vi "UPQLTY.vi"(0 "工位追溯码":string, 1 "检测项目":string, 2 "单位":string, 3 "检测值":string, 4 "检测结果":string, 5 "错误输入":errorcluster, 6 "总成追溯码":string, 7 "设备编号":string, 8 "操作员":string, 9 "产品型号":string, 11 "标准值":string) -> (19 "error out":errorcluster)   [LabVIEW 2020]
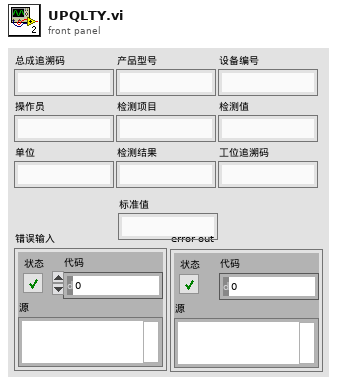
[diagram p1: front panel]
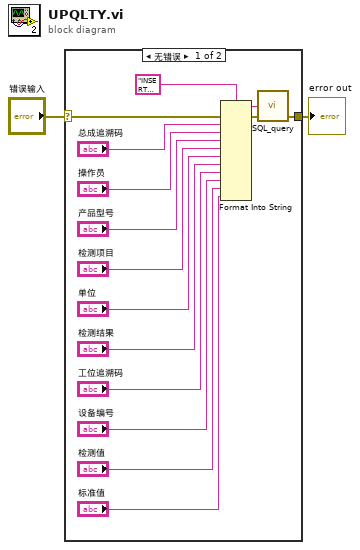
[diagram p0: block diagram]
diagram:
  n1 = case shown="无错误" "错误输入" {
    selector: "错误输入" -> [w5 w18]
    tunnel: [w4 w18] -> w1
    frame No Error {
      n2 = Format Into String(format string="INSERT INTO [SanliServer].[dbo].[产品质量2] (\n\t[总成追溯码],\n\t[操作员],\n\t[产品型号],\n\t[检测项目],\n\t[单位],\n\t[检测结果],\n\t[工位追溯码],\n\t[设备编号],\n\t[检测值],\n [标准值]\n)VALUES\n\t(\n\t\tN'%s',\n\t\tN'%s',\n\t\tN'%s',\n\t\tN'%s',\n\t\tN'%s',\n\t\tN'%s',\n\t\tN'%s',\n\t\tN'%s',\n\t\tN'%s',\n  N'%s'\n\t)", error in=w5, "总成追溯码", "操作员", "产品型号", "检测项目", "单位", "检测结果", "工位追溯码", "设备编号", "检测值", "标准值") -> (resulting string=w7:string, error out=w6:errorcluster)  [unwired: 1 in]
      n3 = call "SQL_query.vi"("error in (no error)"=w6, "SQL query"=w7) -> ("error out"=w4:errorcluster)  [unwired: 1 in, 2 out]
    }
    frame Error {
    }
  }
  "error out" <- w1
